vi "Initial Target Angle Immediate Wrapper.vi"() -> ()   [LabVIEW 2019]
panel:
  in  "Target Real Angle":dbl
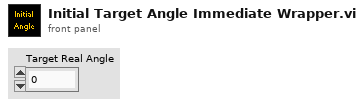
[diagram p1: front panel]
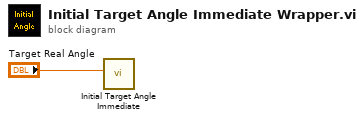
[diagram p0: block diagram]
diagram:
  n1 = call "Initial Target Angle Immediate.vi"("Target Real Angle"="Target Real Angle") -> ()  [unwired: 11 in]
